vi "putRobotClosestPositionInHeadOfArray.vi"(8 "id to not consider in search":i32=-1, 9 "RobotRef":refnum<class "Robot.lvclass">[](array[class]), 10 "position":dbl[](array[numeric]) format="%#_13g", 11 "Utilities in":refnum<class "Utilities.lvclass">) -> (2 "robotId closest Point":i32, 3 "RobotRef out":refnum<class "Robot.lvclass">[](array[class]))   [LabVIEW 2020, in "Ally.lvclass"]
uses:
  Ally.lvclass
  Robot_class/Robot.lvclass
  Utilities_class/Utilities.lvclass
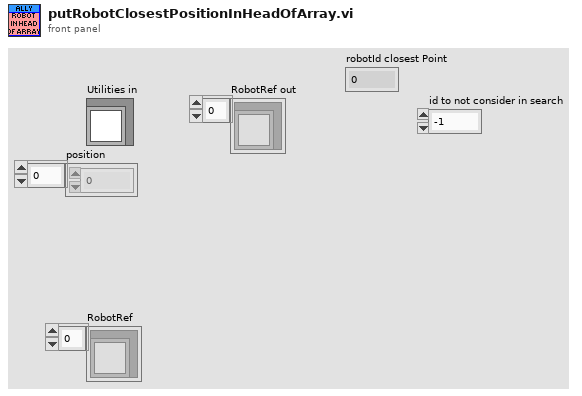
[diagram p1: front panel]
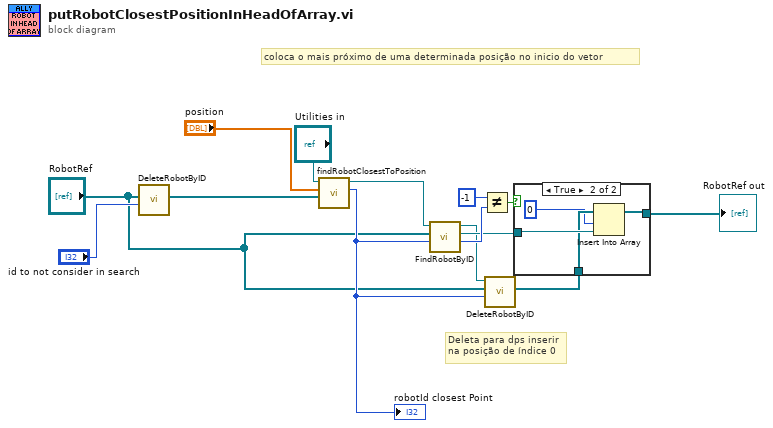
[diagram p0: block diagram]
diagram:
  # "Deleta para dps inserir\nna posição de índice 0"
  # "coloca o mais próximo de uma determinada posição no inicio do vetor"
  n1 = call "DeleteRobotByID.vi"("id"="id to not consider in search", "RobotRef"="RobotRef") -> ("RobotRef out"=w2:refnum<class "Robot.lvclass">[])  [unwired: 7 in, 2 out]
  n2 = call "findRobotClosestToPosition.vi"("robotsArray"=w2, "position"="position", "Utilities in"="Utilities in") -> ("id"=w5:i32, "Utilities out"=w14:refnum<class "Utilities.lvclass">)  [unwired: 5 in, 2 out]
  "robotId closest Point" <- w5
  n3 = call "FindRobotByID.vi"("id"=w5, "RobotRef"="RobotRef", "Utilities in"=w14) -> ("index"=w10:i32, "Robot"=w7:refnum<class "Robot.lvclass">, "Utilities out"=w6:refnum<class "Utilities.lvclass">)  [unwired: 5 in, 1 out]
  n4 = Not Equal?(x=-1, y=w10) -> (x != y?=w12:bool)
  n5 = call "DeleteRobotByID.vi"("id"=w5, "RobotRef"="RobotRef", "Utilities in"=w6) -> ("RobotRef out"=w9:refnum<class "Robot.lvclass">[])  [unwired: 6 in, 2 out]
  n6 = case shown="True" w12 {
    tunnel: w7 -> [_ w19]
    tunnel: [w15 w18] -> w8
    tunnel: w9 -> [w15 w17]
    frame False {
    }
    frame True {
      n7 = Insert Into Array(array=w17, index=0, new element=w19) -> (w18:refnum<class "Robot.lvclass">[])
    }
  }
  "RobotRef out" <- w8
